vi "Get Processes Lookup.vi"(11 "Process in":refnum<class "Process.lvclass">) -> (2 "Processes Lookup":T1[](array[typedef]), 3 "Process out":refnum<class "Process.lvclass">)   [LabVIEW 2019, in "TimingDRV Engine.lvlib" / "Process.lvclass"]
uses:
  Process.lvclass
  TypeDefs/Process Lookup.ctl
  TypeDefs/Message.ctl
  TypeDefs/Update.ctl
  Process.lvclass/Process.ctl
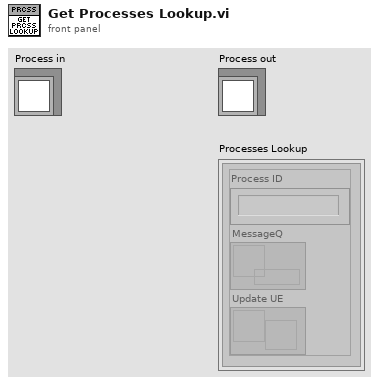
[diagram p1: front panel]
types:
  T1 = typedef "TimingDRV Engine.lvlib/Process.lvclass/Process Lookup.ctl" = cluster{"Process ID":string, "MessageQ":refnum<queue>, "Update UE":refnum<user-event>}
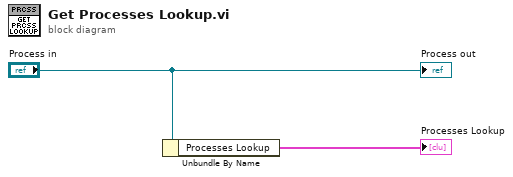
[diagram p0: block diagram]
diagram:
  n1 = Unbundle By Name("Process in") -> ("Processes Lookup"=→"Processes Lookup":T1[])
  "Process out" <- "Process in"
